vi "Check to end beam.vi"(7 "Index":i32, 10 "Current Array":T4[](array[typedef]), 11 "Archive Array":T4[](array[typedef])) -> (2 "Current Array Out":T4[](array[typedef]), 3 "Archive Array Out":T4[](array[typedef]), 5 "Set Transfered Out":set{T1}(c389))   [LabVIEW 2023]
uses:
  Map_Order.ctl
  Cluster_Tracking point.ctl
  Cluster_Point.ctl
  ENUM_Direction_a2.ctl
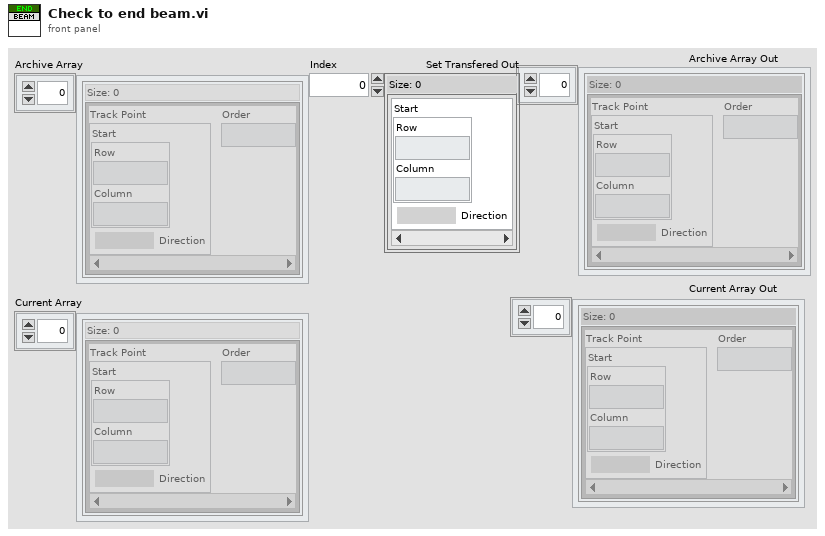
[diagram p1: front panel]
types:
  T1 = typedef "Cluster_Tracking point.ctl" = cluster{"Start":T2, "Direction":T3}
  T2 = typedef "Cluster_Point.ctl" = cluster{"Row":i32, "Column":i32}
  T3 = typedef "ENUM_Direction_a2.ctl" = enum16{"Up", "Left", "Down", "Right", "Up-Down", "Left-Right"}
  T4 = typedef "Map_Order.ctl" = map{T1, i32}
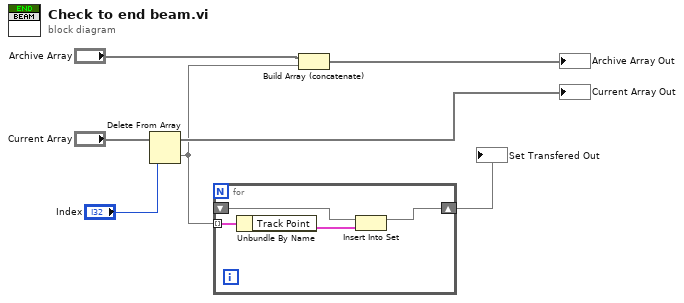
[diagram p0: block diagram]
diagram:
  n1 = Delete From Array(array="Current Array", index="Index") -> (deleted portion=w2:T4, array with subset deleted=→"Current Array Out":T4[])  [unwired: 1 in]
  n2 = for {
    tunnel: w2 -> [w11] mode=indexing
    shift-right: [w9] -> w3
    shift-left: _ -> [w8]
    n3 = Unbundle By Name(w11) -> ("Track Point"=w10:T1)
    n4 = Insert Into Set(10:w10, 11:w8) -> (3:w9:set{T1})  [unwired: 1 out]
  }
  "Set Transfered Out" <- w3
  n5 = Build Array (concatenate)("Archive Array", w2) -> (→"Archive Array Out":T4[])
